vi "CODMn通讯.vi"() -> ()   [LabVIEW 2016, in "斯坦道CODMn新电路板.lvlib"]
uses:
  <vilib>/NI/Modbus Library/API/Wrapper/Create TCP Slave.vi
  <vilib>/Utility/config.llb/Write Key (String).vi
  <vilib>/Plasmionique/MB Master/MB_Master/MB_Master.lvclass
  <vilib>/NI/Modbus Library/API/Slave/Modbus Slave.lvclass
  <vilib>/Utility/config.llb/NI_LVConfig.lvlib
  <vilib>/Plasmionique/MB Master/MB Master.lvlib
  <vilib>/NI/Modbus Library/API/Wrapper/API Main.lvlib
panel:
  out "控制命令 2":u16[](array[numeric]) format="%xH"
  out "状态告警区":T1 {"工作状态" items=["空闲"=0, "水样测试"=1, "标样核查"=2, "零点核查"=3, "跨度核查"=4, "空白测试"=5, "平行样测试"=6, "加标回收"=7, "空白校准"=8, "标样校准"=9, "初始化（清洗）"=10, "调试"=22, "填充管路"=30, "清洗管路"=31, "清洗反应杯"=32]; "告警代码" items=["无告警", "缺试剂告警", "缺水样告警", "缺蒸馏水告警", "缺标液告警", "仪表漏液告警", "标定异常告警", "超量程告警", "加热异常", "低试剂预警", "超上限告警", "超下限告警", "仪表内部其他异常", "滴定异常告警", "电极异常告警", "量程切换告警", "参数设置告警", "PH电极电位异常", "电导率电极异常", "浊度光度异常", "溶解氧电极异常", "溶解氧光强异常", "温度异常告警", "PH异常告警", "溶解氧异常告警", "电导率异常告警", "浊度异常告警", "叶绿素异常告警", "藻密度异常告警", "蓝绿藻异常告警", "ORP异常告警", "氨氮异常告警", "清洁刷异常告警", "SD卡异常告警", "蓝牙异常告警", "Wifi异常告警", "流程异常告警"]; "故障代码" items=["无故障", "电机故障", "温度故障", "通讯故障", "滴定故障"]}
  out "测量数据区":T2 {"单位" items=["ug/L", "mg/L", "ppm", "mg/m3", "cm", "ppb", "ug/m3", "%", "nmol/mol", "umol/mol", "MPN/L", "MPN/100ml", "ng/m3", "NTU", "无量纲", "ms/cm", "us/cm", "℃", "mV", "万个/L"]}
  out "状态告警区":u16[](array[numeric])
  out "测量数据区":u16[](array[numeric])
  out "序列号":string
  out "status":bool
  out "关键参数区":T3
  in  "读关键参数区":bool
  in  "读状态告警区":bool
  in  "读测量数据区":bool
  in  "站号":u16(ring) items=["CODMn"=21, "氨氮"=3]
  in  "停止":bool
  in  "启动":bool
  in  "控制命令":u16(ring) items=["启动测量"=1, "标样核查"=2, "零点核查"=3, "跨度核查"=4, "空白测试"=5, "平行样测试"=6, "加标回收"=7, "空白校准"=8, "标样校准"=9, "初始化（清洗）"=10, "停止测试"=11, "仪器重启"=12, "校时"=13, "模式设置"=14, "测量间隔设置"=15]
  in  "控制命令参数":u16[](array[numeric]) format="%04xH"
  in  "VISA Resource":refnum<visa-resource-name>
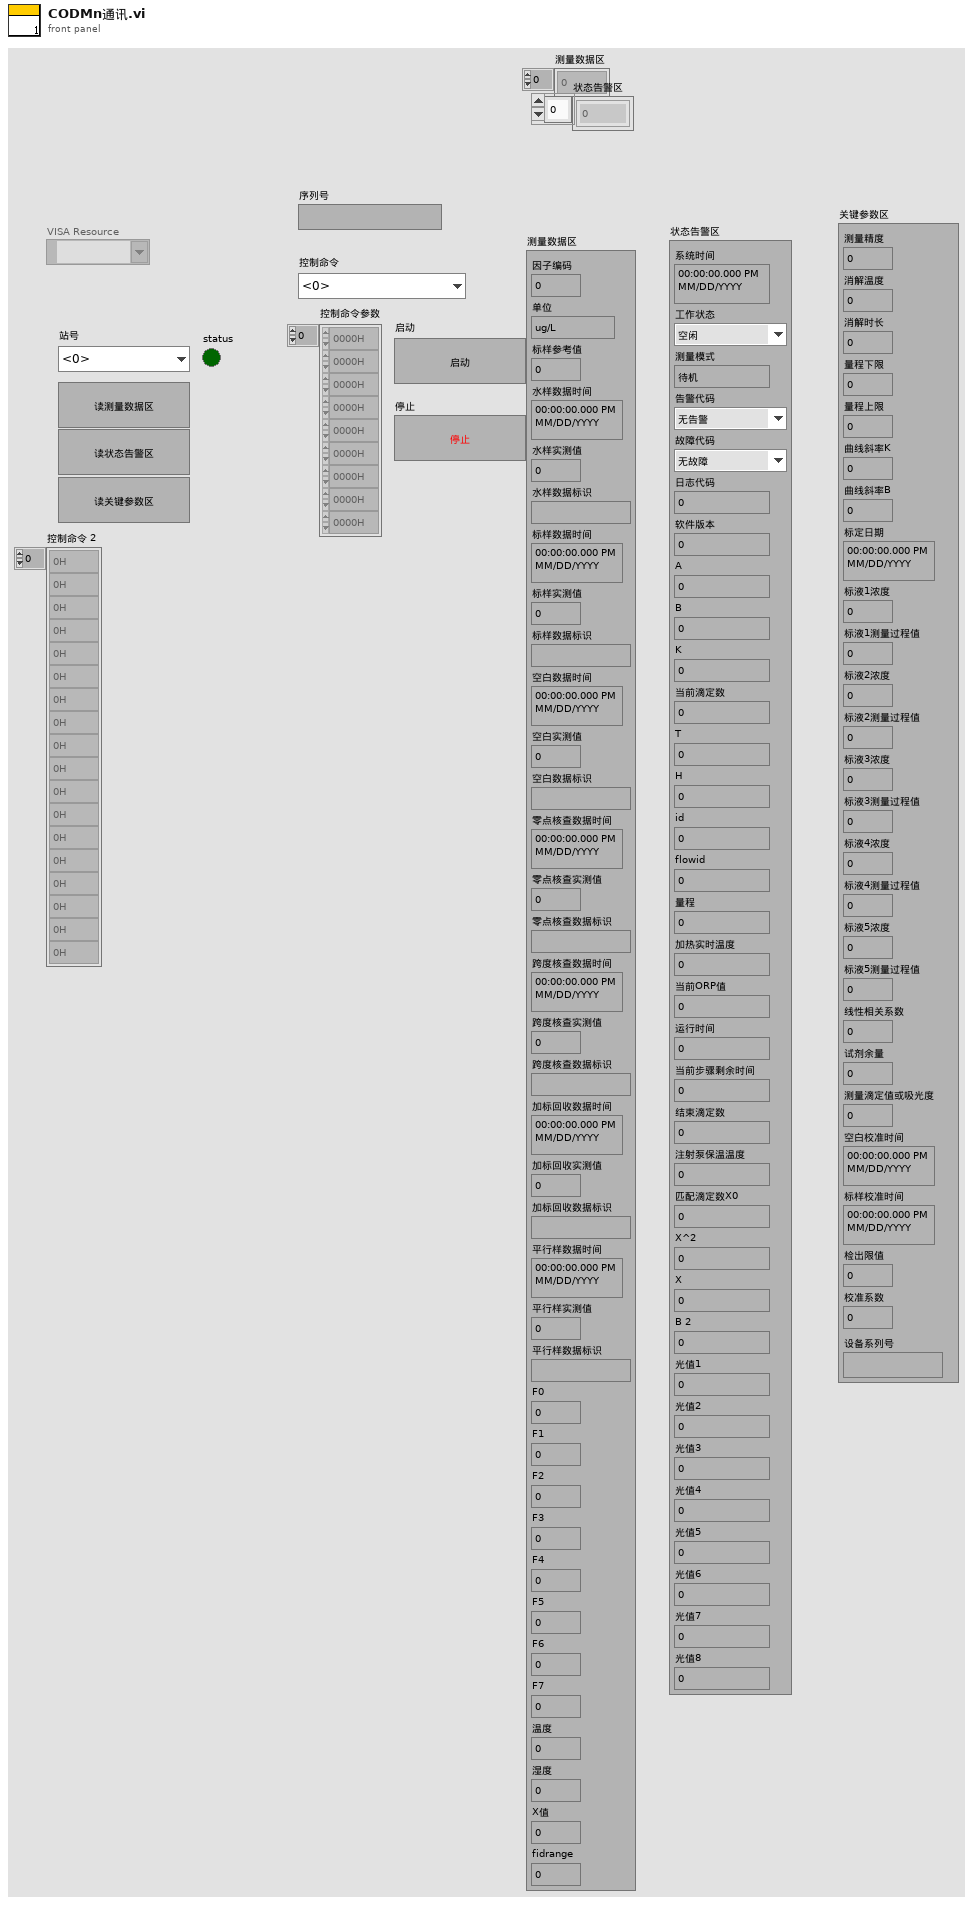
[diagram p1: front panel]
types:
  T1 = cluster{"系统时间":timestamp, "工作状态":u16, "测量模式":enum16{"待机", "连续模式", "周期模式", "定点模式", "受控模式", "手动模式"}, "告警代码":u16, "故障代码":u16, "日志代码":u16, "软件版本":u16, "A":sgl, "B":sgl, "K":sgl, "当前滴定数":sgl, "T":sgl, "H":sgl, "id":u16, "flowid":u16, "量程":u16, "加热实时温度":sgl, "当前ORP值":sgl, "运行时间":sgl, "当前步骤剩余时间":sgl, "结束滴定数":sgl, "注射泵保温温度":sgl, "匹配滴定数X0":u16, "X^2":sgl, "X":sgl, "B 2":sgl, "光值1":sgl, "光值2":sgl, "光值3":sgl, "光值4":sgl, "光值5":sgl, "光值6":sgl, "光值7":sgl, "光值8":sgl}
  T2 = cluster{"因子编码":u32, "单位":u16, "标样参考值":sgl, "水样数据时间":timestamp, "水样实测值":sgl, "水样数据标识":string, "标样数据时间":timestamp, "标样实测值":sgl, "标样数据标识":string, "空白数据时间":timestamp, "空白实测值":sgl, "空白数据标识":string, "零点核查数据时间":timestamp, "零点核查实测值":sgl, "零点核查数据标识":string, "跨度核查数据时间":timestamp, "跨度核查实测值":sgl, "跨度核查数据标识":string, "加标回收数据时间":timestamp, "加标回收实测值":sgl, "加标回收数据标识":string, "平行样数据时间":timestamp, "平行样实测值":sgl, "平行样数据标识":string, "F0":sgl, "F1":sgl, "F2":sgl, "F3":sgl, "F4":sgl, "F5":sgl, "F6":sgl, "F7":sgl, "温度":sgl, "湿度":sgl, "X值":sgl, "fidrange":sgl}
  T3 = cluster{"测量精度":u16, "消解温度":u16, "消解时长":u16, "量程下限":sgl, "量程上限":sgl, "曲线斜率K":sgl, "曲线斜率B":sgl, "标定日期":timestamp, "标液1浓度":sgl, "标液1测量过程值":sgl, "标液2浓度":sgl, "标液2测量过程值":sgl, "标液3浓度":sgl, "标液3测量过程值":sgl, "标液4浓度":sgl, "标液4测量过程值":sgl, "标液5浓度":sgl, "标液5测量过程值":sgl, "线性相关系数":sgl, "试剂余量":u32, "测量滴定值或吸光度":sgl, "空白校准时间":timestamp, "标样校准时间":timestamp, "检出限值":sgl, "校准系数":sgl, "设备系列号":string}
  T4 = typedef "CODMn交互.ctl" = cluster{"COD浓度（mg/L)":dbl, "水样启动时间":timestamp, "加标回收启动时间":timestamp, "CODMn工作状态":enum16{"空闲", "水样测试", "标样核查", "零点核查", "跨度核查", "空白测试", "平行样测试", "加标回收", "空白校准", "标样校准", "初始化（清洗）"}, "多列列表框":i32, "平台试剂余量百分比":sgl, "关键参数":cluster{"测量量程":dbl, "测量精度":dbl, "测量间隔":dbl, "消解温度":dbl, "消解时长":dbl, "空白校准时间":timestamp, "曲线截距":dbl, "曲线斜率":dbl, "测量检出限":dbl, "测量信号值":dbl, "线性相关系数":dbl, "二次多项式系数":dbl, "标样校准时间":timestamp, "稀释倍数":dbl, "三项式系数":dbl, "空白标定系数":dbl, "量程系数":dbl, "F0/ORPA":dbl, "F1/ORPB":dbl, "F2/ORPK":dbl, "F3":dbl, "F4":dbl, "F5":dbl, "F6":dbl, "F7":dbl, "X0/滴定数":dbl, "量程":dbl}, "关键参数改变":bool, "校准信息":cluster{"低标液1浓度":dbl, "低标液1信号值":dbl, "低标液1启用":u16, "低标液2浓度":dbl, "低标液2信号值":dbl, "低标液2启用":u16, "低标液3浓度":dbl, "低标液3信号值":dbl, "低标液3启用":u16, "低标液4浓度":dbl, "低标液4信号值":dbl, "低标液4启用":u16, "低标液5浓度":dbl, "低标液5信号值":dbl, "低标液5启用":u16, "高标液1浓度":dbl, "高标液1信号值":dbl, "高标液1启用":u16, "高标液2浓度":dbl, "高标液2信号值":dbl, "高标液2启用":u16, "高标液3浓度":dbl, "高标液3信号值":dbl, "高标液3启用":u16, "高标液4浓度":dbl, "高标液4信号值":dbl, "高标液4启用":u16, "高标液5浓度":dbl, "高标液5信号值":dbl, "高标液5启用":u16, "低斜率":dbl, "低截距":dbl, "低二次多项式系数":dbl, "低线性相关系数":dbl, "高斜率":dbl, "高截距":dbl, "高二次多项式系数":dbl, "高线性相关系数":dbl}, "校准信息改变":bool, "固件版本号":string}
  T5 = cluster{"测量模式":enum16{"水样测量", "标样核查", "零点核查", "跨度核查", "空白测试", "加标回收", "平行样", "校零", "校标"}}
  T6 = typedef "NI_LVConfig.lvlib/Config Data RefNum.ctl" = refnum<k1>
  T7 = typedef "量程选择控件.ctl" = enum32{"L", "H", "AUTO"}
  T8 = cluster{"水样测试量程模式":T7, "标样核查量程模式":T7, "零点核查量程模式":T7, "跨度核查量程模式":T7, "空白测试量程模式":T7, "平行样测试量程模式":T7, "加标回收量程模式":T7, "空白校准量程模式":T7, "标样校准量程模式":T7}
  T9 = cluster{"测量量程":dbl, "测量精度":dbl, "测量间隔":dbl, "消解温度":dbl, "消解时长":dbl, "空白校准时间":timestamp, "曲线截距":dbl, "曲线斜率":dbl, "测量检出限":dbl, "测量信号值":dbl, "线性相关系数":dbl, "二次多项式系数":dbl, "标样校准时间":timestamp, "稀释倍数":dbl, "三项式系数":dbl, "空白标定系数":dbl, "量程系数":dbl, "F0/ORPA":dbl, "F1/ORPB":dbl, "F2/ORPK":dbl, "F3":dbl, "F4":dbl, "F5":dbl, "F6":dbl, "F7":dbl, "X0/滴定数":dbl, "量程":dbl}
  T10 = cluster{"低标液1浓度":dbl, "低标液1信号值":dbl, "低标液1启用":u16, "低标液2浓度":dbl, "低标液2信号值":dbl, "低标液2启用":u16, "低标液3浓度":dbl, "低标液3信号值":dbl, "低标液3启用":u16, "低标液4浓度":dbl, "低标液4信号值":dbl, "低标液4启用":u16, "低标液5浓度":dbl, "低标液5信号值":dbl, "低标液5启用":u16, "高标液1浓度":dbl, "高标液1信号值":dbl, "高标液1启用":u16, "高标液2浓度":dbl, "高标液2信号值":dbl, "高标液2启用":u16, "高标液3浓度":dbl, "高标液3信号值":dbl, "高标液3启用":u16, "高标液4浓度":dbl, "高标液4信号值":dbl, "高标液4启用":u16, "高标液5浓度":dbl, "高标液5信号值":dbl, "高标液5启用":u16, "低斜率":dbl, "低截距":dbl, "低二次多项式系数":dbl, "低线性相关系数":dbl, "高斜率":dbl, "高截距":dbl, "高二次多项式系数":dbl, "高线性相关系数":dbl}
  T11 = cluster{"站号":u16, "量程切换":enum32{"H", "L", "AUTO"}, "控制命令":u16, "模式设置":enum16{"待机", "连续模式", "周期模式", "定点模式", "受控模式", "手动模式"}, "测量间隔":u16}
  T12 = enum16{"水样测量", "标样核查", "零点核查", "跨度核查", "空白测试", "加标回收", "平行样", "校零", "校标"}
  T13 = enum8{"Enabled", "Disabled", "Disabled and Grayed Out"}
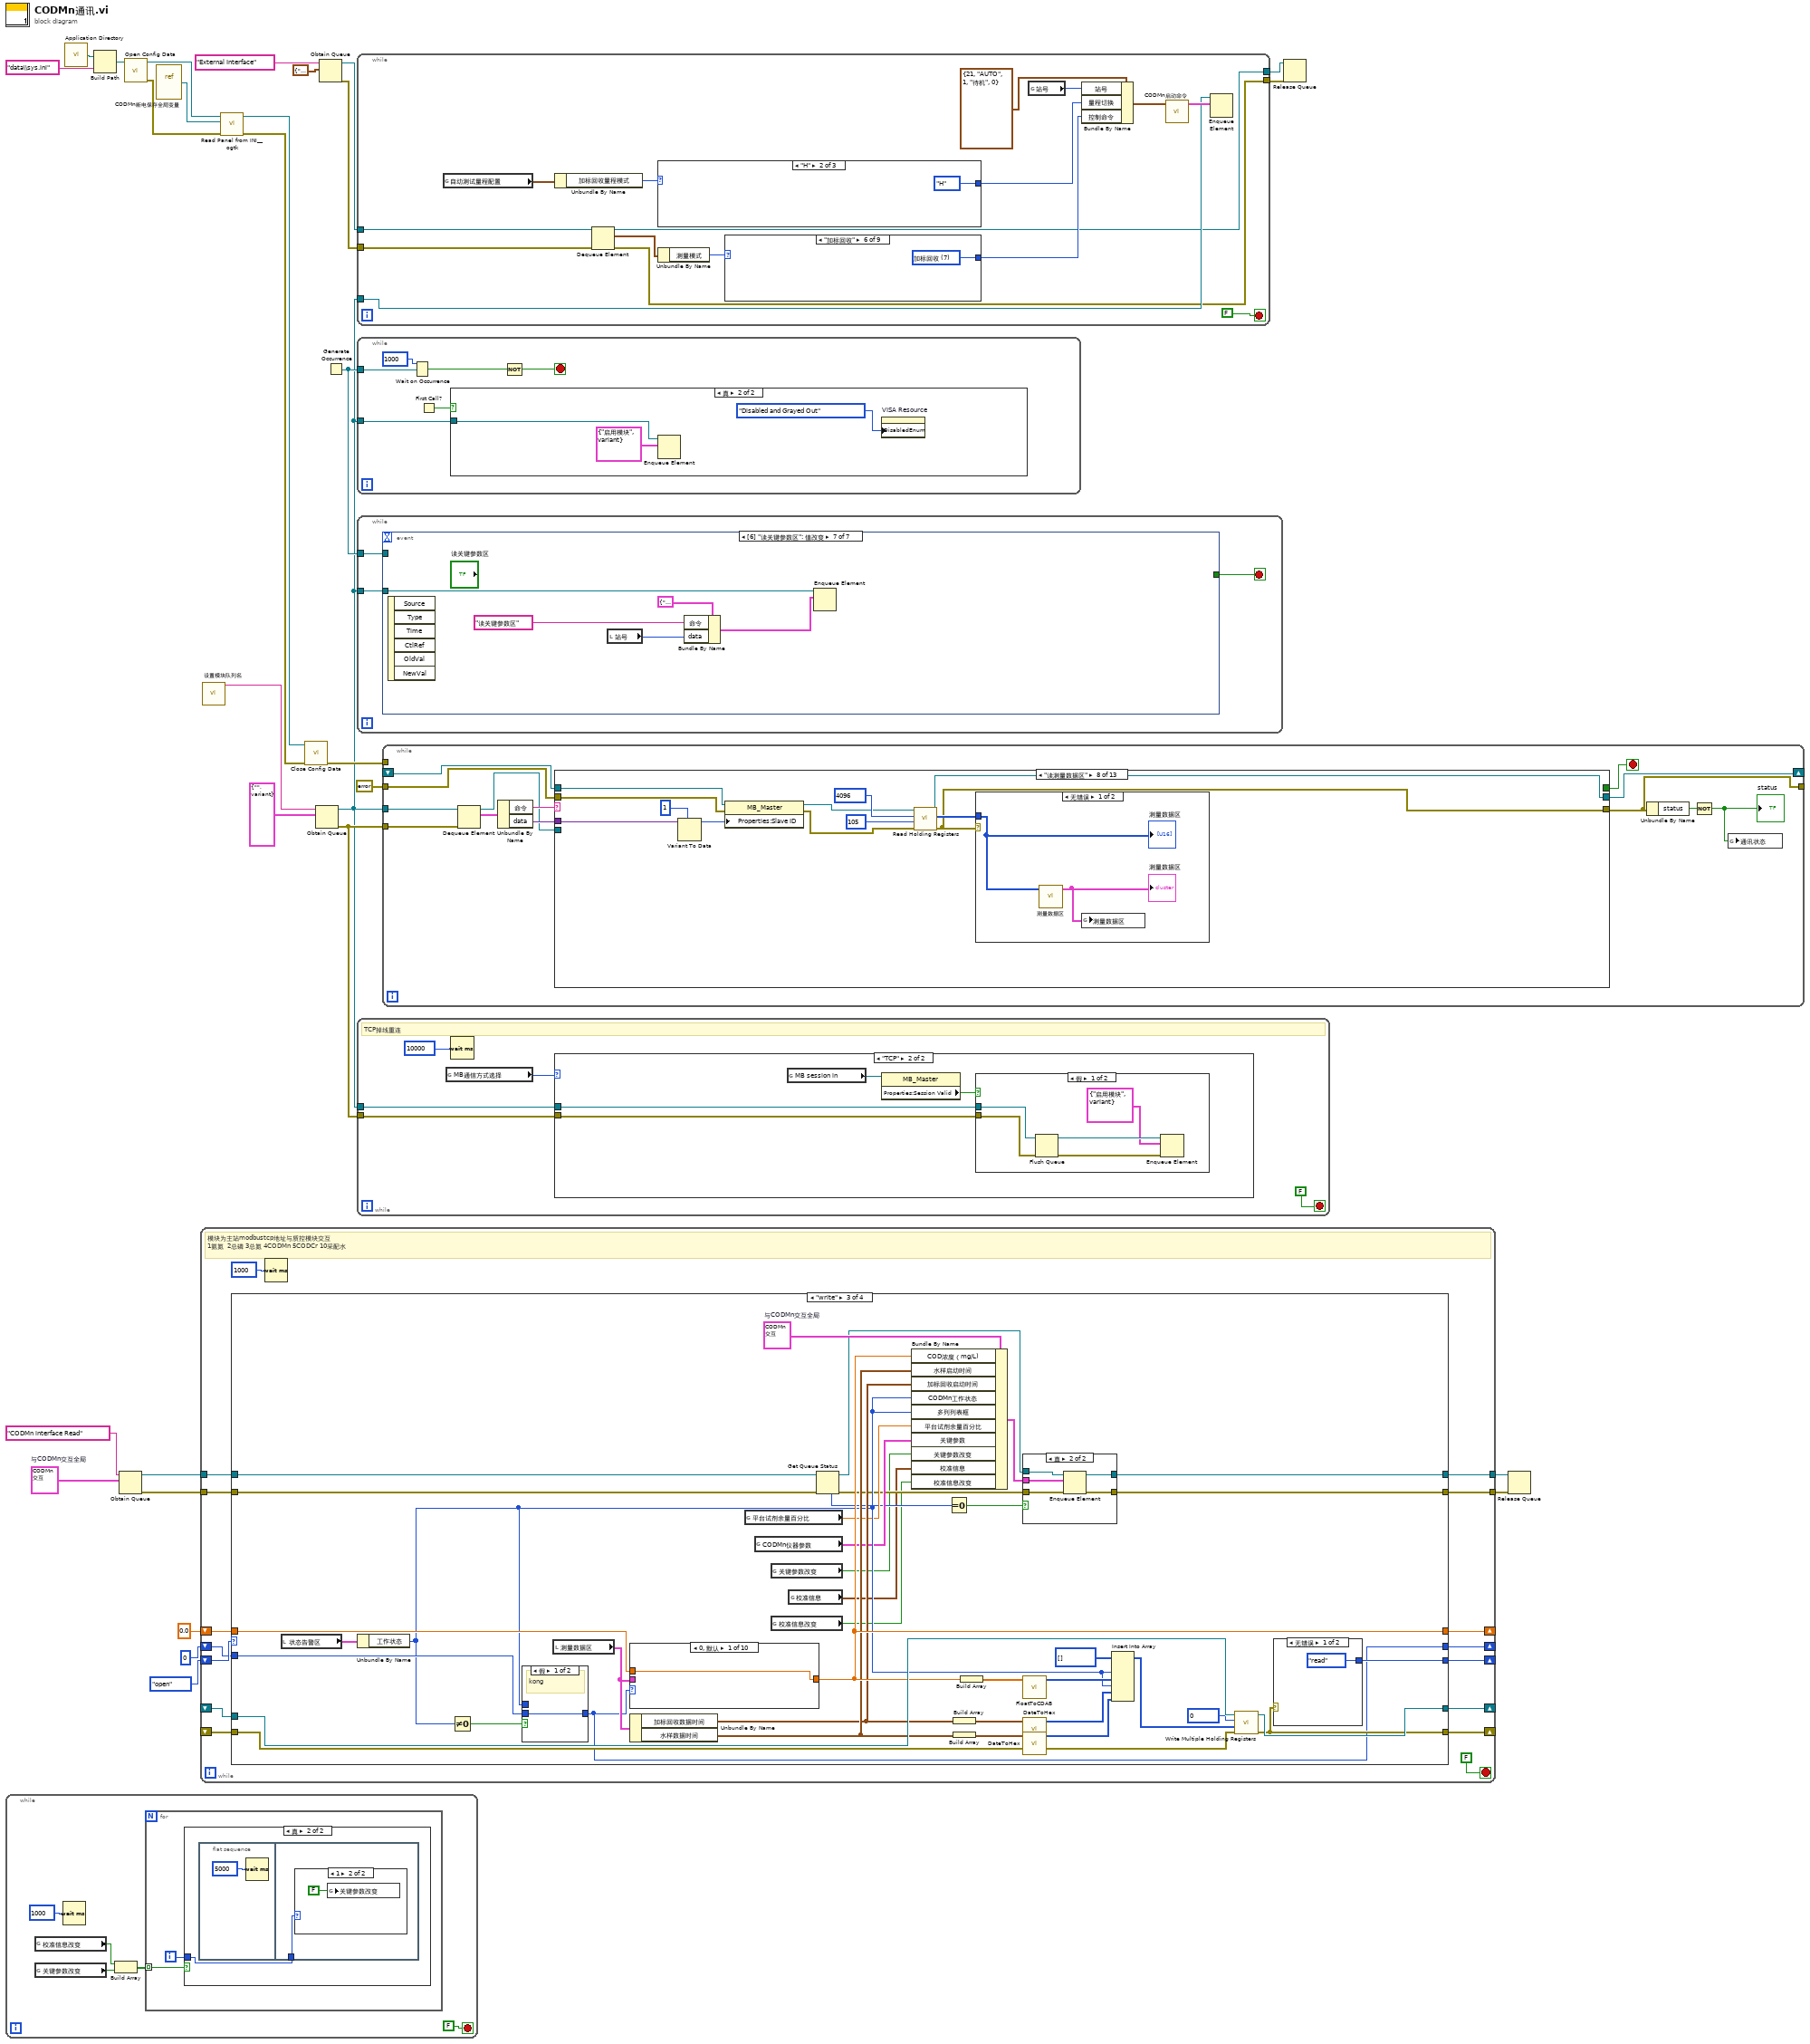
[diagram p0: block diagram]
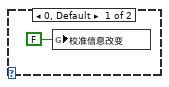
[diagram p3: hidden frame]
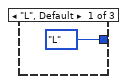
[diagram p4: hidden frame]
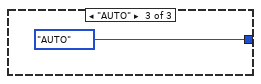
[diagram p5: hidden frame]
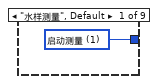
[diagram p6: hidden frame]
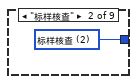
[diagram p7: hidden frame]
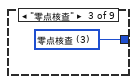
[diagram p8: hidden frame]
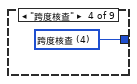
[diagram p9: hidden frame]
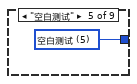
[diagram p10: hidden frame]
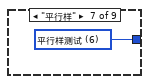
[diagram p11: hidden frame]
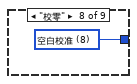
[diagram p12: hidden frame]
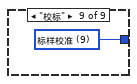
[diagram p13: hidden frame]
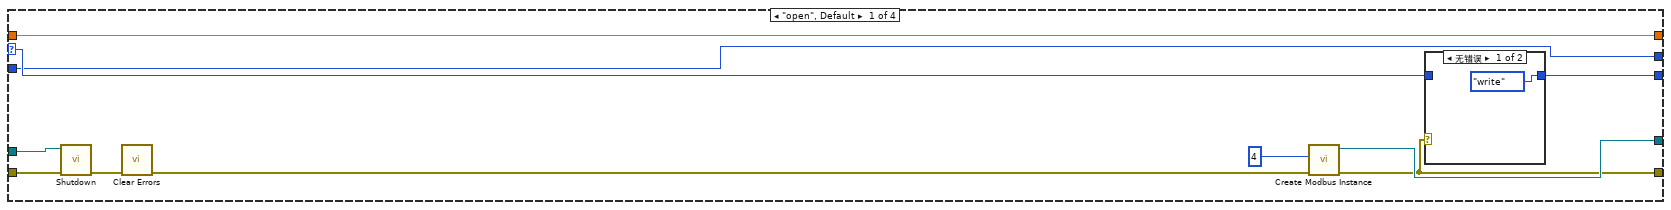
[diagram p16: hidden frame]
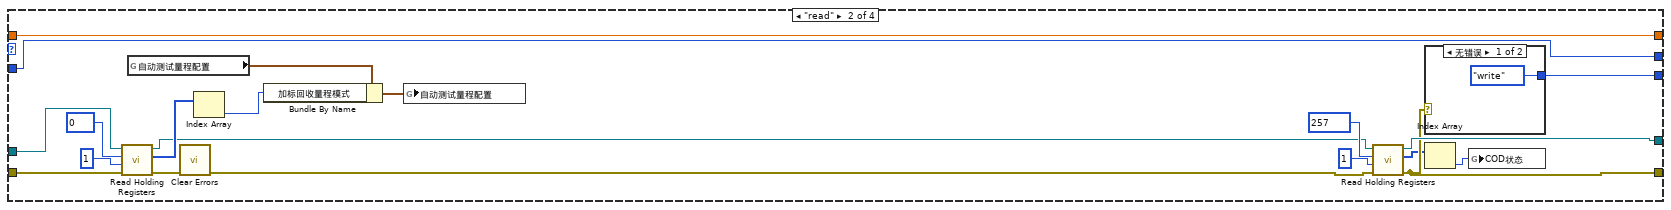
[diagram p18: hidden frame]
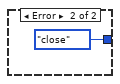
[diagram p19: hidden frame]
diagram:
  w7 = T4 {"COD浓度（mg/L)"=0.0, "水样启动时间"=timestamp(0 s since 1904-01-01), "加标回收启动时间"=timestamp(0 s since 1904-01-01), "CODMn工作状态"=enum."空闲", "多列列表框"=0, "平台试剂余量百分比"=0.0, "关键参数"={"测量量程"=0.0, "测量精度"=0.0, "测量间隔"=0.0, "消解温度"=0.0, "消解时长"=0.0, "空白校准时间"=timestamp(0 s since 1904-01-01), "曲线截距"=0.0, "曲线斜率"=0.0, "测量检出限"=0.0, "测量信号值"=0.0, "线性相关系数"=0.0, "二次多项式系数"=0.0, "标样校准时间"=timestamp(0 s since 1904-01-01), "稀释倍数"=0.0, "三项式系数"=0.0, "空白标定系数"=0.0, "量程系数"=0.0, "F0/ORPA"=0.0, "F1/ORPB"=0.0, "F2/ORPK"=0.0, "F3"=0.0, "F4"=0.0, "F5"=0.0, "F6"=0.0, "F7"=0.0, "X0/滴定数"=0.0, "量程"=0.0}, "关键参数改变"=FALSE, "校准信息"={"低标液1浓度"=0.0, "低标液1信号值"=0.0, "低标液1启用"=0, "低标液2浓度"=0.0, "低标液2信号值"=0.0, "低标液2启用"=0, "低标液3浓度"=0.0, "低标液3信号值"=0.0, "低标液3启用"=0, "低标液4浓度"=0.0, "低标液4信号值"=0.0, "低标液4启用"=0, "低标液5浓度"=0.0, "低标液5信号值"=0.0, "低标液5启用"=0, "高标液1浓度"=0.0, "高标液1信号值"=0.0, "高标液1启用"=0, "高标液2浓度"=0.0, "高标液2信号值"=0.0, "高标液2启用"=0, "高标液3浓度"=0.0, "高标液3信号值"=0.0, "高标液3启用"=0, "高标液4浓度"=0.0, "高标液4信号值"=0.0, "高标液4启用"=0, "高标液5浓度"=0.0, "高标液5信号值"=0.0, "高标液5启用"=0, "低斜率"=0.0, "低截距"=0.0, "低二次多项式系数"=0.0, "低线性相关系数"=0.0, "高斜率"=0.0, "高截距"=0.0, "高二次多项式系数"=0.0, "高线性相关系数"=0.0}, "校准信息改变"=FALSE, "固件版本号"=""}  # 与CODMn交互全局
  n1 = while {
    stop <- FALSE stop-if-true
    n2 = global read "CODMn断电保存全局变量.vi" "校准信息改变"() -> (w33:bool)
    n3 = global read "CODMn断电保存全局变量.vi" "关键参数改变"() -> (w32:bool)
    n4 = Wait (ms)(milliseconds to wait=u32 1000 ("等待时间（毫秒）")) -> ()  [unwired: 1 out]
    n5 = Build Array(w33, w32) -> (w31:bool[])
    n6 = for {
      tunnel: w31 -> [w37] mode=indexing
      i -> [w36]
      n7 = case shown="真" w37 {
        tunnel: w36 -> [_ w38]
        frame False {
        }
        frame True {
          n8 = flat-sequence {
            tunnel: w38 -> [w40]
            frame #0 {
              n9 = Wait (ms)(milliseconds to wait=u32 5000 ("等待时间（毫秒）")) -> ()  [unwired: 1 out]
            }
            frame #1 {
              n10 = case shown="1" w40 {
                frame 0, Default {
                  n11 = global write "CODMn断电保存全局变量.vi" "校准信息改变"(FALSE ("关键参数改变")) -> ()
                }
                frame 1 {
                  n12 = global write "CODMn断电保存全局变量.vi" "关键参数改变"(FALSE ("关键参数改变")) -> ()
                }
              }
            }
          }
        }
      }
    }
  }
  n13 = call <vilib>:"Application Directory.vi"() -> ("Application Directory"=w2:path)
  n14 = Build Path(base path=w2, name or relative path="data\\sys.ini" ("名称或相对路径")) -> (appended path=w19:path)
  n15 = Obtain Queue(name (unnamed)="CODMn interface Read" ("写入方名称"), element data type=w7) -> (queue out=w9:refnum<queue>, error out=w4:errorcluster)  [unwired: 3 in, 1 out]
  n16 = call <vilib>:"Open Config Data.vi"("configuration file path"=w19) -> ("error out"=w26:errorcluster, "refnum"=w23:T6)  [unwired: 8 in, 1 out]
  n17 = vi-ref "CODMn断电保存全局变量.vi"() -> (w24:refnum<vi>)
  n18 = while {
    shift-right: [w56] -> _
    shift-left: _ -> [w58]
    shift-right: [w55] -> _
    shift-left: _ -> [w57]
    shift-right: [w52] -> _
    shift-left: enum16{"open", "read", "write", "close"}."open" -> [w53]
    shift-right: [w50] -> _
    shift-left: sgl 0.0 ("标样实测值") -> [w49]
    shift-right: [w48] -> _
    shift-left: u16 0 ("工作状态") -> [w47]
    tunnel: w9 -> [w46]
    tunnel: [w45] -> w6
    tunnel: [w44] -> w5
    tunnel: w4 -> [w43]
    stop <- FALSE stop-if-true
    # "模块为主站modbustcp地址与质控模块交互\n1氨氮  2总磷 3总氮 4CODMn 5CODCr 10采配水"
    n19 = case shown="\"write\"" w53 {
      selector: w53 -> [w69 _ _ _]
      tunnel: w58 -> [w63 w79 w131 w167]
      tunnel: w57 -> [w62 w78 w130 w166]
      tunnel: [w66 w90 w128 w167] -> w56
      tunnel: [w65 w89 w127 w169] -> w55
      tunnel: [w68 w91 w132 enum16{"open", "read", "write", "close"}."open"] -> w52
      tunnel: [w60 w84 w111 w164] -> w50
      tunnel: w49 -> [w60 w84 w124 w164]
      tunnel: [w59 w83 w115 w163] -> w48
      tunnel: w47 -> [w59 w83 w114 w163]
      tunnel: w46 -> [_ _ w105 _]
      tunnel: [_ _ w103 _] -> w45
      tunnel: [_ _ w102 _] -> w44
      tunnel: w43 -> [_ _ w98 _]
      frame "open", Default {
        n20 = call-dynamic "Shutdown.vi"("error in"=w62, "Modbus slave in"=w63) -> ("error out"=w61:errorcluster)  [unwired: 9 in]
        n21 = call <vilib>:"Clear Errors.vi"("error in (no error)"=w61) -> ("error out"=w64:errorcluster)  [unwired: 5 in, 1 out]
        n22 = call-poly <vilib>:"Create Modbus Instance.vi"("error in"=w64, "port (502)"=u16 4) -> ("error out"=w65:errorcluster, "TCP slave instance"=w66:refnum<class "Modbus Slave.lvclass">)  [unwired: 8 in]
        n23 = case shown="无错误" w65 {
          tunnel: w69 -> [_ w71]
          tunnel: [enum16{"open", "read", "write", "close"}."write" w71] -> w68
          frame No Error {
          }
          frame Error {
          }
        }
      }
      frame "read" {
        n24 = call-dynamic <vilib>:"Read Holding Registers.vi"("error in"=w78, "number of inputs"=u16 1, "starting address"=u16 0, "Modbus slave in"=w79) -> ("error out"=w77:errorcluster, "register values"=w82:u16[], "Modbus slave out"=w76:refnum<class "Modbus Slave.lvclass">)  [unwired: 5 in]
        n25 = global read "CODMn断电保存全局变量.vi" "自动测试量程配置"() -> (w74:T8)
        n26 = call <vilib>:"Clear Errors.vi"("error in (no error)"=w77) -> ("error out"=w72:errorcluster)  [unwired: 5 in, 1 out]
        n27 = Index Array(array=w82) -> (element=w73:u16)  [unwired: 1 in]
        n28 = Bundle By Name(cluster=w74, "加标回收量程模式"=w73) -> (w75:T8)
        n29 = global write "CODMn断电保存全局变量.vi" "自动测试量程配置"(w75) -> ()
        n30 = call-dynamic <vilib>:"Read Holding Registers.vi"("error in"=w72, "number of inputs"=u16 1, "starting address"=u16 257, "Modbus slave in"=w76) -> ("error out"=w89:errorcluster, "register values"=w86:u16[], "Modbus slave out"=w90:refnum<class "Modbus Slave.lvclass">)  [unwired: 5 in]
        n31 = case shown="无错误" w89 {
          tunnel: [enum16{"open", "read", "write", "close"}."write" enum16{"open", "read", "write", "close"}."close"] -> w91
          frame No Error {
          }
          frame Error {
          }
        }
        n32 = Index Array(array=w86) -> (element=w85:u16)  [unwired: 1 in]
        n33 = global write "VARCODMn全局变量.vi" "COD状态"(w85) -> ()
      }
      frame "write" {
        w112 = T4 {"COD浓度（mg/L)"=0.0, "水样启动时间"=timestamp(0 s since 1904-01-01), "加标回收启动时间"=timestamp(0 s since 1904-01-01), "CODMn工作状态"=enum."空闲", "多列列表框"=0, "平台试剂余量百分比"=0.0, "关键参数"={"测量量程"=0.0, "测量精度"=0.0, "测量间隔"=0.0, "消解温度"=0.0, "消解时长"=0.0, "空白校准时间"=timestamp(0 s since 1904-01-01), "曲线截距"=0.0, "曲线斜率"=0.0, "测量检出限"=0.0, "测量信号值"=0.0, "线性相关系数"=0.0, "二次多项式系数"=0.0, "标样校准时间"=timestamp(0 s since 1904-01-01), "稀释倍数"=0.0, "三项式系数"=0.0, "空白标定系数"=0.0, "量程系数"=0.0, "F0/ORPA"=0.0, "F1/ORPB"=0.0, "F2/ORPK"=0.0, "F3"=0.0, "F4"=0.0, "F5"=0.0, "F6"=0.0, "F7"=0.0, "X0/滴定数"=0.0, "量程"=0.0}, "关键参数改变"=FALSE, "校准信息"={"低标液1浓度"=0.0, "低标液1信号值"=0.0, "低标液1启用"=0, "低标液2浓度"=0.0, "低标液2信号值"=0.0, "低标液2启用"=0, "低标液3浓度"=0.0, "低标液3信号值"=0.0, "低标液3启用"=0, "低标液4浓度"=0.0, "低标液4信号值"=0.0, "低标液4启用"=0, "低标液5浓度"=0.0, "低标液5信号值"=0.0, "低标液5启用"=0, "高标液1浓度"=0.0, "高标液1信号值"=0.0, "高标液1启用"=0, "高标液2浓度"=0.0, "高标液2信号值"=0.0, "高标液2启用"=0, "高标液3浓度"=0.0, "高标液3信号值"=0.0, "高标液3启用"=0, "高标液4浓度"=0.0, "高标液4信号值"=0.0, "高标液4启用"=0, "高标液5浓度"=0.0, "高标液5信号值"=0.0, "高标液5启用"=0, "低斜率"=0.0, "低截距"=0.0, "低二次多项式系数"=0.0, "低线性相关系数"=0.0, "高斜率"=0.0, "高截距"=0.0, "高二次多项式系数"=0.0, "高线性相关系数"=0.0}, "校准信息改变"=FALSE, "固件版本号"=""}  # 与CODMn交互全局
        n34 = local read "状态告警区"() -> (w113:T1)
        n35 = Unbundle By Name(w113) -> ("工作状态"=w108:u16)
        n36 = Not Equal To 0?(x=w108) -> (x != 0?=w116:bool)
        n37 = case shown="假" w116 {
          tunnel: w108 -> [_ w141]
          tunnel: [w140 w141] -> w115
          tunnel: w114 -> [w140 _]
          frame False {
            # "kong"
          }
          frame True {
            # "..."
          }
        }
        n38 = local read "测量数据区"() -> (w121:T2)
        n39 = case shown="0, 默认" w115 {
          tunnel: [w142 w144 w146 w148 w150 w152 w154 w156 w158 w160] -> w111
          tunnel: w124 -> [w142 _ _ _ _ _ _ _ _ _]
          tunnel: w121 -> [_ w143 w145 w147 w149 w151 w153 w155 w157 w159]
          frame 0, Default {
          }
          frame 1 {
            n40 = Unbundle By Name(w143) -> ("水样实测值"=w144:sgl)
          }
          frame 2 {
            n41 = Unbundle By Name(w145) -> ("标样实测值"=w146:sgl)
          }
          frame 3 {
            n42 = Unbundle By Name(w147) -> ("零点核查实测值"=w148:sgl)
          }
          frame 4 {
            n43 = Unbundle By Name(w149) -> ("跨度核查实测值"=w150:sgl)
          }
          frame 5 {
            n44 = Unbundle By Name(w151) -> ("空白实测值"=w152:sgl)
          }
          frame 6 {
            n45 = Unbundle By Name(w153) -> ("平行样实测值"=w154:sgl)
          }
          frame 7 {
            n46 = Unbundle By Name(w155) -> ("加标回收实测值"=w156:sgl)
          }
          frame 8 {
            n47 = Unbundle By Name(w157) -> ("空白实测值"=w158:sgl)
          }
          frame 9 {
            n48 = Unbundle By Name(w159) -> ("标样实测值"=w160:sgl)
          }
        }
        n49 = Unbundle By Name(w121) -> ("加标回收数据时间"=w109:timestamp, "水样数据时间"=w110:timestamp)
        n50 = global read "VARCODMn全局变量.vi" "平台试剂余量百分比"() -> (w107:sgl)
        n51 = global read "CODMn断电保存全局变量.vi" "CODMn仪器参数"() -> (w106:T9)
        n52 = global read "CODMn断电保存全局变量.vi" "关键参数改变"() -> (w96:bool)
        n53 = global read "CODMn断电保存全局变量.vi" "校准信息改变"() -> (w94:bool)
        n54 = global read "CODMn断电保存全局变量.vi" "校准信息"() -> (w95:T10)
        n55 = Get Queue Status(queue=w105, error in (no error)=w98) -> (queue out=w101:refnum<queue>, error out=w97:errorcluster, # elements in queue=w100:i32)  [unwired: 1 in, 5 out]
        n56 = Bundle By Name(cluster=w112, "COD浓度（mg/L)"=w111, "水样启动时间"=w110, "加标回收启动时间"=w109, "CODMn工作状态"=w108, "多列列表框"=w108, "平台试剂余量百分比"=w107, "关键参数"=w106, "关键参数改变"=w96, "校准信息"=w95, "校准信息改变"=w94) -> (w104:T4)
        n57 = Equal To 0?(x=w100) -> (x = 0?=w99:bool)
        n58 = Build Array(w109) -> (w120:timestamp[])
        n59 = Build Array(w110) -> (w118:timestamp[])
        n60 = Build Array(w111) -> (w123:sgl[])
        n61 = case shown="真" w99 {
          tunnel: w101 -> [w134 w139]
          tunnel: w104 -> [_ w138]
          tunnel: [w134 w137] -> w103
          tunnel: [w133 w136] -> w102
          tunnel: w97 -> [w133 w135]
          frame False {
          }
          frame True {
            n62 = Enqueue Element(queue=w139, element=w138, error in (no error)=w135) -> (queue out=w137:refnum<queue>, error out=w136:errorcluster)  [unwired: 1 in, 1 out]
          }
        }
        n63 = call "FloatToCDAB.vi"("浮点数"=w123) -> ("CDAB整形输出"=w122:u16[])  [unwired: 10 in]
        n64 = call "DateToHex.vi"("DATE"=w120) -> ("数组"=w119:u16[])  [unwired: 10 in]
        n65 = call "DateToHex.vi"("DATE"=w118) -> ("数组"=w117:u16[])  [unwired: 10 in]
        n66 = Insert Into Array(array=u16[] [] ("values"), new element #1=w108, new element #2=w122, new element #3=w108, new element #4=w119, new element #5=w117) -> (w125:u16[])  [unwired: 1 in]
        n67 = call-dynamic "Write Multiple Holding Registers.vi"("error in"=w130, "registers to write"=w125, "starting address"=u16 0, "Modbus slave in"=w131) -> ("error out"=w127:errorcluster, "Modbus slave out"=w128:refnum<class "Modbus Slave.lvclass">)  [unwired: 6 in]
        n68 = case shown="无错误" w127 {
          tunnel: [enum16{"open", "read", "write", "close"}."read" enum16{"open", "read", "write", "close"}."close"] -> w132
          frame No Error {
          }
          frame Error {
          }
        }
      }
      frame "close" {
        n69 = call-dynamic "Shutdown.vi"("error in"=w166, "Modbus slave in"=w167) -> ("error out"=w165:errorcluster)  [unwired: 9 in]
        n70 = call <vilib>:"Clear Errors.vi"("error in (no error)"=w165) -> ("error out"=w169:errorcluster)  [unwired: 5 in, 1 out]
      }
    }
    n71 = Wait (ms)(milliseconds to wait=u32 1000 ("等待时间（毫秒）")) -> ()  [unwired: 1 out]
  }
  n72 = call "设置模块队列名.vi"() -> ("Msg"=w3:string)  [unwired: 11 in]
  n73 = call <userlib>:"Read Panel from INI__ogtk.vi"("error in (no error)"=w26, "VI ref"=w24, "refnum"=w23) -> ("error out"=w27:errorcluster, "refnum out"=w25:T6)  [unwired: 7 in]
  n74 = call <vilib>:"Close Config Data.vi"("error in (no error)"=w27, "refnum"=w25) -> ("error out"=w22:errorcluster)  [unwired: 8 in, 1 out]
  n75 = Obtain Queue(name (unnamed)=w3, element data type=cluster{"命令":string, "data":variant} {"命令"="", "data"=variant}) -> (queue out=w14:refnum<queue>, error out=w20:errorcluster)  [unwired: 3 in, 1 out]
  n76 = Obtain Queue(name (unnamed)="External Interface" ("名称（未命名）"), element data type=T5 {"测量模式"=enum."水样测量"} ("元素")) -> (queue out=w16:refnum<queue>, error out=w15:errorcluster)  [unwired: 3 in, 1 out]
  n77 = Generate Occurrence() -> (w28:refnum<k4>)
  n78 = while {
    tunnel: w16 -> [w185]
    tunnel: w15 -> [w184]
    tunnel: w14 -> [w176]
    tunnel: [w175] -> w13
    tunnel: [w174] -> w12
    stop <- FALSE stop-if-true
    n79 = global read "CODMn断电保存全局变量.vi" "自动测试量程配置"() -> (w172:T8)
    n80 = Unbundle By Name(w172) -> ("加标回收量程模式"=w171:T7)
    n81 = Dequeue Element(queue=w185, error in (no error)=w184) -> (queue out=w175:refnum<queue>, element=w179:T5, error out=w174:errorcluster)  [unwired: 1 in, 1 out]
    n82 = case shown="\"H\"" w171 {
      tunnel: [enum32{"H", "L", "AUTO"}."L" ("量程切换") enum32{"H", "L", "AUTO"}."H" ("量程切换") enum32{"H", "L", "AUTO"}."AUTO" ("量程切换")] -> w170
      frame "L", Default {
      }
      frame "H" {
      }
      frame "AUTO" {
      }
    }
    n83 = Unbundle By Name(w179) -> ("测量模式"=w178:T12)
    n84 = case shown="\"加标回收\"" w178 {
      tunnel: [w189 w190 w191 w192 w193 w194 w195 w196 w197] -> w177
      frame "水样测量", Default {
        w189 = u16 1 items=["启动测量"=1, "标样核查"=2, "零点核查"=3, "跨度核查"=4, "空白测试"=5, "平行样测试"=6, "加标回收"=7, "空白校准"=8, "标样校准"=9, "初始化（清洗）"=10, "停止测试"=11, "仪器重启"=12, "校时"=13, "模式设置"=14, "测量间隔设置"=15, "调试"=22, "填充管路"=30, "清洗管路"=31, "清洗反应杯"=32] ("控制命令")
      }
      frame "标样核查" {
        w190 = u16 2 items=["启动测量"=1, "标样核查"=2, "零点核查"=3, "跨度核查"=4, "空白测试"=5, "平行样测试"=6, "加标回收"=7, "空白校准"=8, "标样校准"=9, "初始化（清洗）"=10, "停止测试"=11, "仪器重启"=12, "校时"=13, "模式设置"=14, "测量间隔设置"=15, "调试"=22, "填充管路"=30, "清洗管路"=31, "清洗反应杯"=32] ("控制命令")
      }
      frame "零点核查" {
        w191 = u16 3 items=["启动测量"=1, "标样核查"=2, "零点核查"=3, "跨度核查"=4, "空白测试"=5, "平行样测试"=6, "加标回收"=7, "空白校准"=8, "标样校准"=9, "初始化（清洗）"=10, "停止测试"=11, "仪器重启"=12, "校时"=13, "模式设置"=14, "测量间隔设置"=15, "调试"=22, "填充管路"=30, "清洗管路"=31, "清洗反应杯"=32] ("控制命令")
      }
      frame "跨度核查" {
        w192 = u16 4 items=["启动测量"=1, "标样核查"=2, "零点核查"=3, "跨度核查"=4, "空白测试"=5, "平行样测试"=6, "加标回收"=7, "空白校准"=8, "标样校准"=9, "初始化（清洗）"=10, "停止测试"=11, "仪器重启"=12, "校时"=13, "模式设置"=14, "测量间隔设置"=15, "调试"=22, "填充管路"=30, "清洗管路"=31, "清洗反应杯"=32] ("控制命令")
      }
      frame "空白测试" {
        w193 = u16 5 items=["启动测量"=1, "标样核查"=2, "零点核查"=3, "跨度核查"=4, "空白测试"=5, "平行样测试"=6, "加标回收"=7, "空白校准"=8, "标样校准"=9, "初始化（清洗）"=10, "停止测试"=11, "仪器重启"=12, "校时"=13, "模式设置"=14, "测量间隔设置"=15, "调试"=22, "填充管路"=30, "清洗管路"=31, "清洗反应杯"=32] ("控制命令")
      }
      frame "加标回收" {
        w194 = u16 7 items=["启动测量"=1, "标样核查"=2, "零点核查"=3, "跨度核查"=4, "空白测试"=5, "平行样测试"=6, "加标回收"=7, "空白校准"=8, "标样校准"=9, "初始化（清洗）"=10, "停止测试"=11, "仪器重启"=12, "校时"=13, "模式设置"=14, "测量间隔设置"=15, "调试"=22, "填充管路"=30, "清洗管路"=31, "清洗反应杯"=32] ("控制命令")
      }
      frame "平行样" {
        w195 = u16 6 items=["启动测量"=1, "标样核查"=2, "零点核查"=3, "跨度核查"=4, "空白测试"=5, "平行样测试"=6, "加标回收"=7, "空白校准"=8, "标样校准"=9, "初始化（清洗）"=10, "停止测试"=11, "仪器重启"=12, "校时"=13, "模式设置"=14, "测量间隔设置"=15, "调试"=22, "填充管路"=30, "清洗管路"=31, "清洗反应杯"=32] ("控制命令")
      }
      frame "校零" {
        w196 = u16 8 items=["启动测量"=1, "标样核查"=2, "零点核查"=3, "跨度核查"=4, "空白测试"=5, "平行样测试"=6, "加标回收"=7, "空白校准"=8, "标样校准"=9, "初始化（清洗）"=10, "停止测试"=11, "仪器重启"=12, "校时"=13, "模式设置"=14, "测量间隔设置"=15, "调试"=22, "填充管路"=30, "清洗管路"=31, "清洗反应杯"=32] ("控制命令")
      }
      frame "校标" {
        w197 = u16 9 items=["启动测量"=1, "标样核查"=2, "零点核查"=3, "跨度核查"=4, "空白测试"=5, "平行样测试"=6, "加标回收"=7, "空白校准"=8, "标样校准"=9, "初始化（清洗）"=10, "停止测试"=11, "仪器重启"=12, "校时"=13, "模式设置"=14, "测量间隔设置"=15, "调试"=22, "填充管路"=30, "清洗管路"=31, "清洗反应杯"=32] ("控制命令")
      }
    }
    n85 = global read "CODMn断电保存全局变量.vi" "站号"() -> (w180:u16)
    n86 = Bundle By Name(cluster=T11 {"站号"=21, "量程切换"=enum."AUTO", "控制命令"=1, "模式设置"=enum."待机", "测量间隔"=0} ("参数"), "站号"=w180, "量程切换"=w170, "控制命令"=w177) -> (w181:T11)
    n87 = call "CODMn启动命令.vi"("参数"=w181) -> ("启动命令"=w183:cluster{"命令":string, "data":variant})  [unwired: 10 in]
    n88 = Enqueue Element(queue=w176, element=w183) -> ()  [unwired: 2 in, 3 out]
  }
  n89 = while {
    tunnel: w28 -> [w203]
    tunnel: w14 -> [w199]
    stop <- w200 stop-if-true
    n90 = Wait on Occurrence(2:w203, 3:1000 ("毫秒超时(-1)")) -> (0:w201:bool)  [unwired: 1 in]
    n91 = First Call?() -> (First Call?: T/F=w198:bool)
    n92 = case shown="真" w198 {
      tunnel: w199 -> [_ w205]
      frame False {
      }
      frame True {
        n93 = Enqueue Element(queue=w205, element=cluster{"命令":string, "data":variant} {"命令"="启用模块", "data"=variant} ("元素")) -> ()  [unwired: 2 in, 3 out]
        n94 = property on="VISA Resource" class="VISAName"("DisabledEnum"=T13."Disabled and Grayed Out" ("禁用")) -> ()  [unwired: 2 in, 2 out]
      }
    }
    n95 = Not(x=w201) -> (.not. x?=w200:bool)
  }
  n96 = while {
    tunnel: w14 -> [w209]
    tunnel: w28 -> [w207]
    stop <- w208 stop-if-true
    n97 = event shown="[6] \"读关键参数区\": 值改变" {
      selector: _ -> [_ _ _ _ _ _ _]
      dyn-events: _ -> [_ _ _ _ _ _ _]
      timeout: _ -> [_ _ _ _ _ _ _]
      tunnel: w209 -> [_ _ w230 w237 w243 w248 w253]
      tunnel: [_ _ _ "停止" _ _ _] -> w208
      tunnel: w207 -> [_ _ _ w234 _ _ _]
      event Timeout {
        n98 = event-data() -> ()  [unwired: 1 in, 3 out]
      }
      event "VISA Resource": Value Change {
        n99 = event-data() -> ()  [unwired: 1 in, 6 out]
        n100 = call <vilib>:"Application Directory.vi"() -> ("Application Directory"=w212:path)
        n101 = Build Path(base path=w212, name or relative path="data\\set.ini" ("名称或相对路径")) -> (appended path=w213:path)
        n102 = call <vilib>:"Open Config Data.vi"("configuration file path"=w213) -> ("error out"=w219:errorcluster, "refnum"=w218:T6)  [unwired: 8 in, 1 out]
        n103 = call-poly <vilib>:"Write Key.vi"("section"="CODMn", "error in (no error)"=w219, "value"="VISA Resource", "key"="串口", "refnum"=w218) -> ("error out"=w215:errorcluster, "refnum out"=w211:T6)  [unwired: 4 in, 1 out]
        n104 = call <vilib>:"Close Config Data.vi"("error in (no error)"=w215, "refnum"=w211) -> ()  [unwired: 8 in, 2 out]
      }
      event "启动": Value Change {
        n105 = event-data() -> ()  [unwired: 1 in, 6 out]
        n106 = case shown="默认" "控制命令" {
          tunnel: "控制命令参数" -> [w232 w233]
          tunnel: [w231 w233] -> w220
          frame Default {
            n107 = call "HexToWord.vi"("数组"=w232) -> ("WORD"=w231:u16[])  [unwired: 10 in]
          }
          frame 13 {
          }
        }
        n108 = Swap Bytes(anything="控制命令") -> (byte swapped=w223:u16)
        n109 = call "控制命令区.vi"("控制命令参数"=w220, "控制命令"=w223) -> ("控制命令"=w226:u16[])  [unwired: 9 in]
        n110 = local read "站号"() -> (w225:u16)
        n111 = Bundle("站号"=w225, "控制命令"=w226) -> (w224:cluster{"站号":u16, "控制命令":u16[]})  [unwired: 1 in]
        n112 = Bundle By Name(cluster=cluster{"命令":string, "data":variant} {"命令"="", "data"=variant} ("元素"), "命令"="启动", "data"=w224) -> (w228:cluster{"命令":string, "data":variant})
        n113 = Enqueue Element(queue=w230, element=w228) -> ()  [unwired: 2 in, 3 out]
      }
      event "停止": Value Change {
        n114 = event-data() -> ()  [unwired: 1 in, 6 out]
        n115 = Set Occurrence(w234) -> ()
        n116 = Flush Queue(queue=w237) -> (queue out=w236:refnum<queue>)  [unwired: 1 in, 2 out]
        n117 = Enqueue Element(queue=w236, element=cluster{"命令":string, "data":variant} {"命令"="shutdown", "data"=variant} ("元素")) -> ()  [unwired: 2 in, 3 out]
      }
      event "读测量数据区": Value Change {
        n118 = event-data() -> ()  [unwired: 1 in, 6 out]
        n119 = Bundle By Name(cluster=cluster{"命令":string, "data":variant} {"命令"="", "data"=variant} ("元素"), "命令"="读测量数据区", "data"="站号") -> (w241:cluster{"命令":string, "data":variant})
        n120 = Enqueue Element(queue=w243, element=w241) -> ()  [unwired: 2 in, 3 out]
      }
      event "读状态告警区": Value Change {
        n121 = event-data() -> ()  [unwired: 1 in, 6 out]
        n122 = local read "站号"() -> (w244:u16)
        n123 = Bundle By Name(cluster=cluster{"命令":string, "data":variant} {"命令"="", "data"=variant} ("元素"), "命令"="读状态告警区", "data"=w244) -> (w246:cluster{"命令":string, "data":variant})
        n124 = Enqueue Element(queue=w248, element=w246) -> ()  [unwired: 2 in, 3 out]
      }
      event "读关键参数区": Value Change {
        n125 = event-data() -> ()  [unwired: 1 in, 6 out]
        n126 = local read "站号"() -> (w249:u16)
        n127 = Bundle By Name(cluster=cluster{"命令":string, "data":variant} {"命令"="", "data"=variant} ("元素"), "命令"="读关键参数区", "data"=w249) -> (w251:cluster{"命令":string, "data":variant})
        n128 = Enqueue Element(queue=w253, element=w251) -> ()  [unwired: 2 in, 3 out]
      }
    }
  }
  n129 = while "While循环" {
    tunnel: w14 -> [w256]
    tunnel: w20 -> [w255]
    stop <- FALSE stop-if-true
    # "TCP掉线重连"
    n130 = global read "CODMn断电保存全局变量.vi" "MB通信方式选择"() -> (w254:enum16{"串口", "TCP"})
    n131 = Wait (ms)(milliseconds to wait=u32 10000 ("等待时间（毫秒）")) -> ()  [unwired: 1 out]
    n132 = case shown="\"TCP\"" w254 {
      tunnel: w256 -> [_ w261]
      tunnel: w255 -> [_ w260]
      frame "串口", Default {
      }
      frame "TCP" {
        n133 = global read "VARCODMn全局变量.vi" "MB session in"() -> (w259:refnum<class "MB_Master.lvclass">)
        n134 = property class="MB_Master"(reference=w259) -> ("Properties:Session Valid"=w262:bool)  [unwired: 1 in, 2 out]
        n135 = case shown="假" w262 {
          tunnel: w261 -> [w265 _]
          tunnel: w260 -> [w264 _]
          frame False {
            n136 = Flush Queue(queue=w265, error in (no error)=w264) -> (queue out=w267:refnum<queue>, error out=w266:errorcluster)  [unwired: 1 out]
            n137 = Enqueue Element(queue=w267, element=cluster{"命令":string, "data":variant} {"命令"="启用模块", "data"=variant} ("元素"), error in (no error)=w266) -> ()  [unwired: 1 in, 3 out]
          }
          frame True {
          }
        }
      }
    }
  }
  n138 = while {
    tunnel: w14 -> [w280]
    tunnel: w20 -> [w279]
    shift-right: [w277] -> _
    shift-left: _ -> [w276]
    tunnel: errorcluster {"status"=FALSE, "code"=0, "source"=""} ("error out") -> [w275]
    tunnel: [w270] -> _
    tunnel: w22 -> [_]
    stop <- w278 stop-if-true
    n139 = Dequeue Element(queue=w280, error in (no error)=w279) -> (queue out=w271:refnum<queue>, element=w273:cluster{"命令":string, "data":variant})  [unwired: 1 in, 2 out]
    n140 = Unbundle By Name(w273) -> ("命令"=w274:string, "data"=w272:variant)
    n141 = case shown="\"读测量数据区\"" w274 {
      tunnel: w272 -> [_ _ _ w299 w310 w327 w339 w348 w358 w374 w389 w406 _]
      tunnel: w271 -> [_ _ _ _ _ _ _ _ _ _ _ _ w461]
      tunnel: [_ _ _ _ _ _ _ _ _ _ _ _ TRUE] -> w278
      tunnel: [w281 w284 w286 w302 w313 w329 w341 w353 w367 w381 w396 w400 w457] -> w277
      tunnel: [w282 w283 w287 w301 w312 w328 w340 w342 w356 w370 w397 w399 w458] -> w270
      tunnel: w276 -> [w281 _ w286 w298 w309 w326 w338 w347 w361 w377 w392 w407 w457]
      tunnel: w275 -> [w282 _ w289 w295 w306 w323 w335 w345 w362 w378 w393 w408 w459]
      frame Default {
      }
      frame "启用模块" {
        n142 = call "MB_api.vi"("STEP"=enum16{"open", "read", "write", "close"}."open") -> ("error out"=w283:errorcluster, "MB session out"=w284:refnum<class "MB_Master.lvclass">)  [unwired: 8 in, 1 out]
        n143 = global write "VARCODMn全局变量.vi" "MB session in"(w284) -> ()
      }
      frame "停用模块" {
        n144 = call-dynamic "Close Session.vi"("error in (no error)"=w289, "MB session in"=w286) -> ("error out"=w288:errorcluster)  [unwired: 9 in]
        n145 = call <vilib>:"Clear Errors.vi"("error in (no error)"=w288) -> ("error out"=w287:errorcluster)  [unwired: 5 in, 1 out]
      }
      frame "启动" {
        n146 = Variant To Data(type=cluster{"站号":u16, "控制命令":u16[]} {"站号"=0, "控制命令"=[]} ("输出簇"), Variant=w299) -> (data=w293:cluster{"站号":u16, "控制命令":u16[]})  [unwired: 1 in, 1 out]
        n147 = Unbundle By Name(w293) -> ("站号"=w292:u16, "控制命令"=w290:u16[])
        n148 = property class="MB_Master"(reference=w298, error in=w295, "Properties:Slave ID"=w292) -> (reference out=w297:refnum<class "MB_Master.lvclass">, error out=w296:errorcluster)
        n149 = Index Array(array=w290) -> (element=w291:u16)  [unwired: 1 in]
        n150 = global write "VARCODMn全局变量.vi" "控制命令"(w291) -> ()
        n151 = call <vilib>:"Write Multiple Registers.vi"("error in (no error)"=w296, "values"=w290, "starting address"=u16 4608, "MB session in"=w297) -> ("error out"=w301:errorcluster, "MB session out"=w302:refnum<class "MB_Master.lvclass">)  [unwired: 6 in]
      }
      frame "盲样测试" {
        n152 = Variant To Data(type=0, Variant=w310) -> (data=w303:i32)  [unwired: 1 in, 1 out]
        n153 = property class="MB_Master"(reference=w309, error in=w306, "Properties:Slave ID"=w303) -> (reference out=w308:refnum<class "MB_Master.lvclass">, error out=w307:errorcluster)
        n154 = case shown="默认" w303 {
          tunnel: [u16[] [] ("values") u16[] [33539, 0] ("values") u16[] [23555, 0] ("values")] -> w305
          frame Default {
          }
          frame 1 {
            # "总磷盲样测试命令"
          }
          frame 3 {
            # "氨氮盲样测试"
          }
        }
        n155 = call <vilib>:"Write Multiple Registers.vi"("error in (no error)"=w307, "values"=w305, "starting address"=u16 24592, "MB session in"=w308) -> ("error out"=w312:errorcluster, "MB session out"=w313:refnum<class "MB_Master.lvclass">)  [unwired: 6 in]
      }
      frame "debug" {
        n156 = Variant To Data(type=cluster{"站号":u16, "控制命令":u16[]} {"站号"=0, "控制命令"=[]} ("输出簇"), Variant=w327) -> (data=w321:cluster{"站号":u16, "控制命令":u16[]})  [unwired: 1 in, 1 out]
        n157 = Unbundle By Name(w321) -> ("站号"=w320:u16, "控制命令"=w318:u16[])
        "控制命令 2" <- w318
        n158 = property class="MB_Master"(reference=w326, error in=w323, "Properties:Slave ID"=w320) -> (reference out=w325:refnum<class "MB_Master.lvclass">, error out=w324:errorcluster)
        n159 = Index Array(array=w318) -> (element=w319:u16)  [unwired: 1 in]
        n160 = global write "VARCODMn全局变量.vi" "控制命令"(w319) -> ()
        n161 = call <vilib>:"Write Multiple Registers.vi"("error in (no error)"=w324, "values"=w318, "starting address"=u16 24594, "MB session in"=w325) -> ("error out"=w328:errorcluster, "MB session out"=w329:refnum<class "MB_Master.lvclass">)  [unwired: 6 in]
      }
      frame "单步控制" {
        n162 = Variant To Data(type=cluster{"站号":u16, "控制命令":u16[]} {"站号"=0, "控制命令"=[]} ("输出簇"), Variant=w339) -> (data=w333:cluster{"站号":u16, "控制命令":u16[]})  [unwired: 1 in, 1 out]
        n163 = Unbundle By Name(w333) -> ("站号"=w332:u16, "控制命令"=w331:u16[])
        n164 = property class="MB_Master"(reference=w338, error in=w335, "Properties:Slave ID"=w332) -> (reference out=w337:refnum<class "MB_Master.lvclass">, error out=w336:errorcluster)
        n165 = call <vilib>:"Write Multiple Registers.vi"("error in (no error)"=w336, "values"=w331, "starting address"=u16 24610, "MB session in"=w337) -> ("error out"=w340:errorcluster, "MB session out"=w341:refnum<class "MB_Master.lvclass">)  [unwired: 6 in]
      }
      frame "读测量数据区" {
        n166 = Variant To Data(type=u8 1 ("Slave ID"), Variant=w348) -> (data=w349:u8)  [unwired: 1 in, 1 out]
        n167 = property class="MB_Master"(reference=w347, error in=w345, "Properties:Slave ID"=w349) -> (reference out=w346:refnum<class "MB_Master.lvclass">, error out=w344:errorcluster)
        n168 = call <vilib>:"Read Holding Registers.vi"("error in (no error)"=w344, "quantity"=u16 105, "starting address"=u16 4096, "MB session in"=w346) -> ("error out"=w342:errorcluster, "Registers"=w343:u16[], "MB session out"=w353:refnum<class "MB_Master.lvclass">)  [unwired: 5 in]
        n169 = case shown="无错误" w342 {
          tunnel: w343 -> [w355 _]
          frame No Error {
            n170 = call "测量数据区.vi"("数组"=w355) -> ("测量数据区"=w354:T2)  [unwired: 10 in]
            "测量数据区" <- w354
            n171 = global write "VARCODMn全局变量.vi" "测量数据区"(w354) -> ()
            "测量数据区" <- w355
          }
          frame Error {
          }
        }
      }
      frame "读状态告警区" {
        n172 = Variant To Data(type=u8 1 ("Slave ID"), Variant=w358) -> (data=w363:u8)  [unwired: 1 in, 1 out]
        n173 = property class="MB_Master"(reference=w361, error in=w362, "Properties:Slave ID"=w363) -> (reference out=w360:refnum<class "MB_Master.lvclass">, error out=w359:errorcluster)
        n174 = call <vilib>:"Read Holding Registers.vi"("error in (no error)"=w359, "quantity"=u16 56, "starting address"=u16 4224, "MB session in"=w360) -> ("error out"=w356:errorcluster, "Registers"=w357:u16[], "MB session out"=w367:refnum<class "MB_Master.lvclass">)  [unwired: 5 in]
        n175 = case shown="无错误" w356 {
          tunnel: w357 -> [w369 _]
          frame No Error {
            n176 = call "状态告警区.vi"("数组"=w369) -> ("状态告警区"=w368:T1)  [unwired: 10 in]
            "状态告警区" <- w368
            n177 = global write "VARCODMn全局变量.vi" "状态告警区"(w368) -> ()
            "状态告警区" <- w369
          }
          frame Error {
          }
        }
      }
      frame "读关键参数区" {
        n178 = Variant To Data(type=u8 1 ("Slave ID"), Variant=w374) -> (data=w372:u8)  [unwired: 1 in, 1 out]
        n179 = property class="MB_Master"(reference=w377, error in=w378, "Properties:Slave ID"=w372) -> (reference out=w376:refnum<class "MB_Master.lvclass">, error out=w375:errorcluster)
        n180 = call <vilib>:"Read Holding Registers.vi"("error in (no error)"=w375, "quantity"=u16 19, "starting address"=u16 4256, "MB session in"=w376) -> ("error out"=w370:errorcluster, "Registers"=w371:u16[], "MB session out"=w381:refnum<class "MB_Master.lvclass">)  [unwired: 5 in]
        n181 = case shown="无错误" w370 {
          tunnel: w371 -> [w383 _]
          frame No Error {
            n182 = call "关键参数区.vi"("数组"=w383) -> ("关键参数区"=w382:T3)  [unwired: 10 in]
            "关键参数区" <- w382
            n183 = global write "VARCODMn全局变量.vi" "关键参数区"(w382) -> ()
          }
          frame Error {
          }
        }
      }
      frame "读序列号" {
        n184 = Variant To Data(type=u8 1 ("Slave ID"), Variant=w389) -> (data=w387:u8)  [unwired: 1 in, 1 out]
        n185 = property class="MB_Master"(reference=w392, error in=w393, "Properties:Slave ID"=w387) -> (reference out=w391:refnum<class "MB_Master.lvclass">, error out=w390:errorcluster)
        n186 = call <vilib>:"Read Holding Registers.vi"("error in (no error)"=w390, "quantity"=u16 6, "starting address"=u16 4, "MB session in"=w391) -> ("error out"=w397:errorcluster, "Registers"=w386:u16[], "MB session out"=w396:refnum<class "MB_Master.lvclass">)  [unwired: 5 in]
        n187 = call "HexToString.vi"("数组"=w386) -> ("STRING"=w385:string[])  [unwired: 10 in]
        n188 = Index Array(array=w385) -> (element=w384:string)  [unwired: 1 in]
        "序列号" <- w384
        n189 = global write "VARCODMn全局变量.vi" "序列号"(w384) -> ()
      }
      frame "读滴定曲线" {
        n190 = Variant To Data(type=u8 1 ("Slave ID"), Variant=w406) -> (data=w404:u8)  [unwired: 1 in, 1 out]
        n191 = property class="MB_Master"(reference=w407, error in=w408, "Properties:Slave ID"=w404) -> (reference out=w402:refnum<class "MB_Master.lvclass">, error out=w401:errorcluster)
        n192 = global read "VARCODMn全局变量.vi" "V5以上版本"() -> (w403:bool)
        n193 = case shown="真" w403 {
          tunnel: w402 -> [w412 w437]
          tunnel: w401 -> [w413 w436]
          tunnel: [w409 w435] -> w398
          tunnel: [w411 w434] -> w400
          tunnel: [w410 w433] -> w399
          frame False {
            n194 = for {
              tunnel: u16[] [120, 120, 120, 120, 32] -> [w428] mode=indexing
              shift-right: [w432] -> _
              shift-left: u16 24599 ("starting address") -> [w429]
              shift-right: [w430] -> w414
              shift-left: u16[] [] ("新元素/子数组") -> [w431]
              tunnel: w412 -> [w427]
              tunnel: w413 -> [w426]
              tunnel: [w425] -> w411
              tunnel: [w424] -> w410
              n195 = Add(x=w429, y=w428) -> (x+y=w432:u16)
              n196 = call <vilib>:"Read Holding Registers.vi"("error in (no error)"=w426, "quantity"=w428, "starting address"=w429, "MB session in"=w427) -> ("error out"=w424:errorcluster, "Registers"=w423:u16[], "MB session out"=w425:refnum<class "MB_Master.lvclass">)  [unwired: 5 in]
              n197 = call "HexToWord.vi"("数组"=w423) -> ("WORD"=w422:u16[])  [unwired: 10 in]
              n198 = Insert Into Array(array=w431, new element=w422) -> (w430:u16[])  [unwired: 1 in]
            }
            n199 = for {
              tunnel: w414 -> [w421] mode=indexing
              tunnel: [w418] -> w409 mode=indexing
              n200 = Divide(x=w421, y=u16 10) -> (x/y=w419:dbl)
              n201 = To Unsigned Word Integer(number=w419) -> (unsigned 16bit integer=w418:u16)
            }
          }
          frame True {
            n202 = for {
              tunnel: u16[] [120, 120, 120, 120, 32] -> [w452] mode=indexing
              shift-right: [w456] -> _
              shift-left: u16 24615 ("starting address") -> [w453]
              shift-right: [w454] -> w438
              shift-left: u16[] [] ("新元素/子数组") -> [w455]
              tunnel: w437 -> [w451]
              tunnel: w436 -> [w450]
              tunnel: [w449] -> w434
              tunnel: [w448] -> w433
              n203 = Add(x=w453, y=w452) -> (x+y=w456:u16)
              n204 = call <vilib>:"Read Holding Registers.vi"("error in (no error)"=w450, "quantity"=w452, "starting address"=w453, "MB session in"=w451) -> ("error out"=w448:errorcluster, "Registers"=w447:u16[], "MB session out"=w449:refnum<class "MB_Master.lvclass">)  [unwired: 5 in]
              n205 = call "HexToWord.vi"("数组"=w447) -> ("WORD"=w446:u16[])  [unwired: 10 in]
              n206 = Insert Into Array(array=w455, new element=w446) -> (w454:u16[])  [unwired: 1 in]
            }
            n207 = for {
              tunnel: w438 -> [w445] mode=indexing
              tunnel: [w442] -> w435 mode=indexing
              n208 = Divide(x=w445, y=u16 5) -> (x/y=w443:dbl)
              n209 = To Unsigned Word Integer(number=w443) -> (unsigned 16bit integer=w442:u16)
            }
          }
        }
        n210 = global write "VARCODMn全局变量.vi" "ORP滴定曲线"(w398) -> ()
        n211 = global write "VARCODMn全局变量.vi" "滴定数-ORP值"(w398) -> ()
      }
      frame "shutdown" {
        n212 = call-dynamic "Close Session.vi"("error in (no error)"=w459, "MB session in"=w457) -> ("error out"=w458:errorcluster)  [unwired: 9 in]
        n213 = Flush Queue(queue=w461) -> (queue out=w460:refnum<queue>)  [unwired: 1 in, 2 out]
        n214 = Release Queue(queue=w460) -> ()  [unwired: 2 in, 3 out]
      }
    }
    n215 = Unbundle By Name(w270) -> ("status"=w269:bool)
    n216 = Not(x=w269) -> (.not. x?=w268:bool)
    "status" <- w268
    n217 = global write "VARCODMn全局变量.vi" "通讯状态"(w268) -> ()
  }
  n218 = Release Queue(queue=w13, error in (no error)=w12) -> ()  [unwired: 1 in, 3 out]
  n219 = Release Queue(queue=w6, error in (no error)=w5) -> ()  [unwired: 1 in, 3 out]
